vi "load config.vi"(8 "error in (no error)":errorcluster, 10 "cfg file name":string="ic_sparc.cfg", 11 "Channel in":refnum<class "Channel.lvclass">) -> (0 "error out":errorcluster, 3 "Channel out":refnum<class "Channel.lvclass">)   [LabVIEW 2018, in "Channel.lvclass"]
uses:
  Channel.lvclass
  Channel.lvclass/Channel.ctl
  Interface/Interface.lvclass/Interface.ctl
  <vilib>/Utility/config.llb/Read Key (String).vi
  Interface/Interface.lvclass
  <vilib>/Utility/config.llb/NI_LVConfig.lvlib
panel:
  out "#FRAMES":u32
  out "EXPTIME":dbl
  out "JSON string":string
  out "output cluster":T1={"ACQUISITION_MODE"=1, "TRIGGER_MODE"=0, "READ_MODE"=4, "PREAMP"=0, "READOUT_RATE"=0, "VERTICAL_SHIFT_SPEED"=3, "EM_MODE"=0, "EM_GAIN"=2, "SHUTTER_MODE"=2, "SHUTTER_TTL"=0, "SHUTTER_OPENNING_TIME"=50, "SHUTTER_CLOSING_TIME"=50, "VBIN"=1, "HBIN"=1, "INITIAL_LINE"=1, "INITIAL_COLUMN"=1, "FINAL_LINE"=1024, "FINAL_COLUMN"=1024, "FRAME_TRANSFER"=FALSE, "VERTICAL_CLOCK_VOLTAGE"=0, "AD_CHANNEL"=0} {"VERTICAL_CLOCK_VOLTAGE" items=["Normal", "+1", "+2", "+3", "+4"]; "SHUTTER_TTL" items=["TTL Low", "TTl High"]; "SHUTTER_MODE" items=["Fully Auto", "OPEN", "CLOSED"]; "EM_MODE" items=["Electron Multiplying", "Conventional"]; "VERTICAL_SHIFT_SPEED" items=["0.6", "1.13", "2.2", "4.33"]; "READOUT_RATE" items=["1 MHz", "10 MHz", "20 MHz", "30 MHz"]; "PREAMP" items=["Gain 1", "Gain 2"]; "READ_MODE" items=["Full Vertical Binning", "Multi-Track", "Random-track", "Single-Track", "Image"]; "TRIGGER_MODE" items=["Internal", "External", "N/A", "N/A", "N/A", "N/A", "External Start"]; "ACQUISITION_MODE" items=["N/A", "Single", "Accumulate", "Kinetic", "Fast Kinetic"]}
  out "value":string
  out "file created?":bool
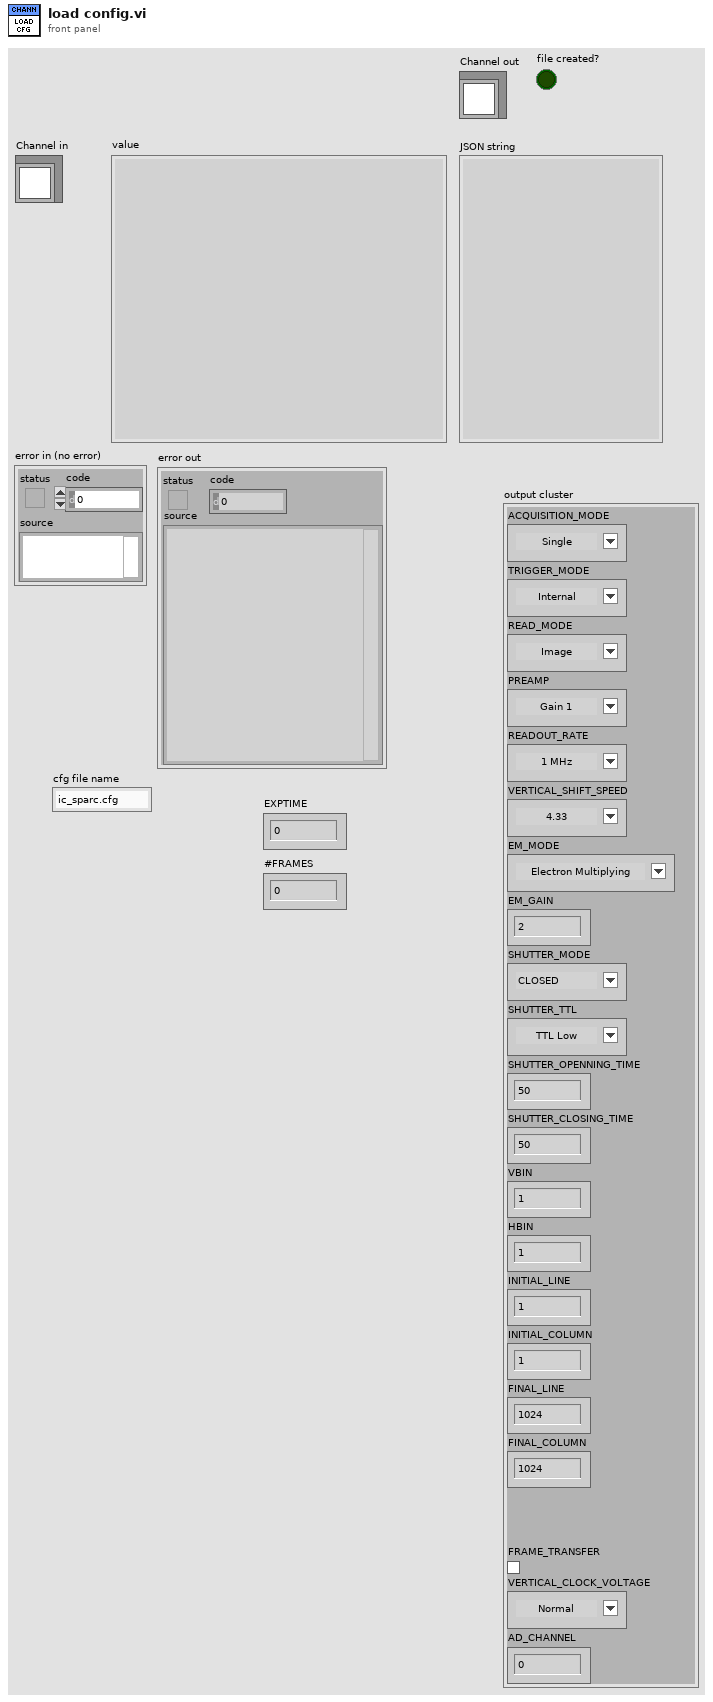
[diagram p1: front panel]
types:
  T1 = cluster{"ACQUISITION_MODE":u8, "TRIGGER_MODE":u8, "READ_MODE":u8, "PREAMP":u8, "READOUT_RATE":u8, "VERTICAL_SHIFT_SPEED":u8, "EM_MODE":u8, "EM_GAIN":u16, "SHUTTER_MODE":u8, "SHUTTER_TTL":u8, "SHUTTER_OPENNING_TIME":u16, "SHUTTER_CLOSING_TIME":u16, "VBIN":u16, "HBIN":u16, "INITIAL_LINE":u16, "INITIAL_COLUMN":u16, "FINAL_LINE":u16, "FINAL_COLUMN":u16, "FRAME_TRANSFER":bool, "VERTICAL_CLOCK_VOLTAGE":u8, "AD_CHANNEL":u32}
  T2 = typedef "NI_LVConfig.lvlib/Config Data RefNum.ctl" = refnum<k1>
  T3 = cluster{"ACQUISITION_MODE":u8, "TRIGGER_MODE":u8, "READ_MODE":u8, "PREAMP":u8, "READOUT_RATE":u8, "VERTICAL_SHIFT_SPEED":u8, "EM_MODE":u8, "EM_GAIN":u16, "SHUTTER_MODE":u8, "SHUTTER_TTL":u8, "SHUTTER_OPENING_TIME":u16, "SHUTTER_CLOSING_TIME":u16, "VBIN":u16, "HBIN":u16, "INITIAL_LINE":u16, "INITIAL_COLUMN":u16, "FINAL_LINE":u16, "FINAL_COLUMN":u16, "FRAME_TRANSFER":bool, "VERTICAL_CLOCK_VOLTAGE":u8, "AD_CHANNEL":u32}
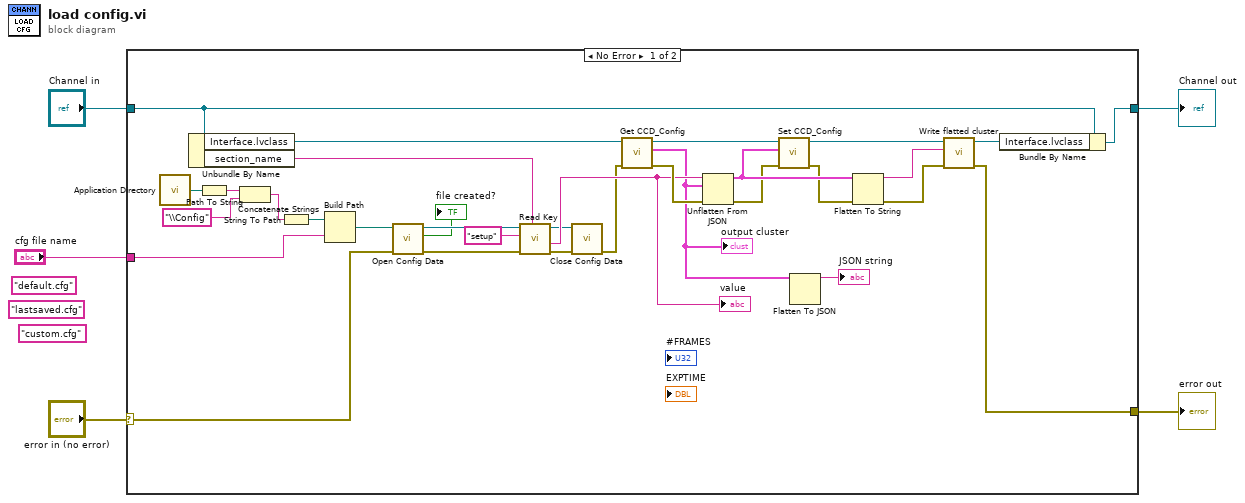
[diagram p0: block diagram]
diagram:
  (unwired) "custom.cfg" ("name or relative path")
  (unwired) "lastsaved.cfg" ("name or relative path")
  (unwired) "default.cfg" ("name or relative path")
  n1 = case shown="No Error" "error in (no error)" {
    selector: "error in (no error)" -> [w31 w39]
    tunnel: [w23 w39] -> w4
    tunnel: [w32 w38] -> w2
    tunnel: "Channel in" -> [w33 w38]
    tunnel: "cfg file name" -> [w11 _]
    frame No Error {
      n2 = call <vilib>:"Application Directory.vi"() -> ("Application Directory"=w10:path)
      n3 = Unbundle By Name(w33) -> ("Interface.lvclass"=w26:refnum<class "Interface.lvclass">, "section_name"=w36:string)
      n4 = Path To String(path=w10) -> (string=w9:string)
      n5 = Concatenate Strings(w9, "\\Config" ("string")) -> (w7:string)
      n6 = String To Path(string=w7) -> (path=w6:path)
      n7 = Build Path(base path=w6, name or relative path=w11) -> (appended path=w37:path)
      n8 = call <vilib>:"Open Config Data.vi"("error in (no error)"=w31, "configuration file path"=w37) -> ("error out"=w25:errorcluster, "file created?"=→"file created?":bool, "refnum"=w35:T2)  [unwired: 7 in]
      n9 = call-poly <vilib>:"Read Key.vi"("section"=w36, "error in (no error)"=w25, "key"="setup", "refnum"=w35) -> ("error out"=w13:errorcluster, "value"=w27:string, "refnum out"=w14:T2)  [unwired: 4 in, 1 out]
      "value" <- w27
      n10 = call <vilib>:"Close Config Data.vi"("error in (no error)"=w13, "refnum"=w14) -> ("error out"=w12:errorcluster)  [unwired: 8 in, 1 out]
      n11 = call-dynamic "Get CCD_Config.vi"("error in (no error)"=w12, "Interface in"=w26) -> ("error out"=w30:errorcluster, "output cluster"=w21:T3, "Interface out"=w18:refnum<class "Interface.lvclass">)  [unwired: 7 in]
      "output cluster" <- w21
      n12 = Unflatten From JSON(JSON string=w27, type and defaults=w21, error in (no error)=w30) -> (value=w19:T3, error out=w17:errorcluster)  [unwired: 4 in]
      n13 = call-dynamic "Set CCD_Config.vi"("error in (no error)"=w17, "output cluster"=w19, "Interface in"=w18) -> ("error out"=w16:errorcluster, "Interface out"=w15:refnum<class "Interface.lvclass">)  [unwired: 7 in]
      n14 = Flatten To JSON(anything=w21) -> (JSON string=→"JSON string":string)  [unwired: 2 in, 1 out]
      n15 = Flatten To String(anything=w19, error in (no error)=w16) -> (data string=w29:string, error out=w28:errorcluster)  [unwired: 2 in, 1 out]
      n16 = call "Write flatted cluster.vi"("error in (no error)"=w28, "flatted cluster"=w29, "Interface in"=w15) -> ("error out"=w23:errorcluster, "Interface out"=w24:refnum<class "Interface.lvclass">)  [unwired: 7 in]
      n17 = Bundle By Name(cluster=w33, "Interface.lvclass"=w24) -> (w32:refnum<class "Channel.lvclass">)
    }
    frame Error {
    }
  }
  "error out" <- w4
  "Channel out" <- w2
